vi "Read IED Measurement Status.vi"(8 "error in (no error)":errorcluster, 11 "IED Measurement Msg in":refnum<class "IED Measurement Status Msg.lvclass">) -> (0 "error out":errorcluster, 1 "Measurement Name":string, 2 "IED Name":string, 3 "IED Measurement Msg out":refnum<class "IED Measurement Status Msg.lvclass">, 4 "Status":T1, 6 "Value/error":string)   [LabVIEW 2015, in "SCADA Core.lvlib" / "IED Measurement Status Msg.lvclass"]
uses:
  IED Measurement Status Msg.lvclass
  IED Measurement Status.ctl
  IED Measurement Status Msg.lvclass/IED Measurement Status Msg.ctl
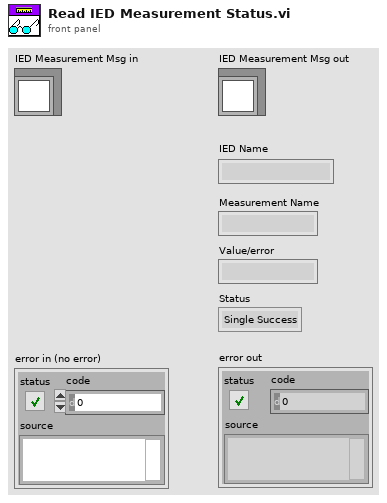
[diagram p1: front panel]
types:
  T1 = typedef "SCADA Core.lvlib/IED Measurement Status Msg.lvclass/IED Measurement Status.ctl" = enum16{"Single Success", "Single Failure", "Multiple Success", "Multiple Failure"}
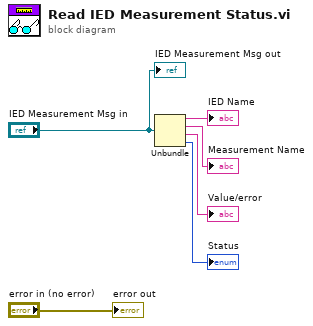
[diagram p0: block diagram]
diagram:
  n1 = Unbundle("IED Measurement Msg in") -> (→"IED Name":string, →"Measurement Name":string, →"Value/error":string, →"Status":T1)
  "IED Measurement Msg out" <- "IED Measurement Msg in"
  "error out" <- "error in (no error)"
